vi "LED flashing 1.vi"(0 "Arduino Resource In":T1={"VISA resource"="", "Board Type"=enum."Uno", "Connection Type"=enum."USB / Serial", "Bytes Per Packet (15)"=15}, 11 "Error Out In":errorcluster, 12 "Текущий раствор":i32) -> (1 "1":bool, 2 "2":bool, 3 "3":bool, 4 "Arduino Resource Out":T1={"VISA resource"="", "Board Type"=enum."Uno", "Connection Type"=enum."USB / Serial", "Bytes Per Packet (15)"=15}, 15 "Error Out":errorcluster)   [LabVIEW 2016]
uses:
  <vilib>/LabVIEW Interface for Arduino/Type Defs/Arduino Resource.ctl
  <vilib>/LabVIEW Interface for Arduino/Type Defs/Board Type.ctl
  <vilib>/LabVIEW Interface for Arduino/LabVIEW Interface for Arduino.lvlib
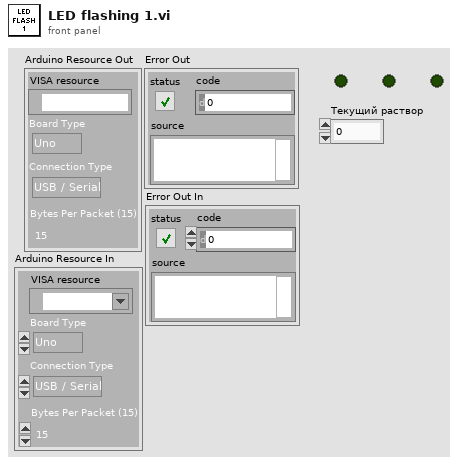
[diagram p1: front panel]
types:
  T1 = typedef "LabVIEW Interface for Arduino.lvlib/Arduino Resource.ctl" = cluster{"VISA resource":refnum<visa-resource-name>, "Board Type":T2, "Connection Type":enum8{"USB / Serial"}, "Bytes Per Packet (15)":u8}
  T2 = typedef "LabVIEW Interface for Arduino.lvlib/Board Type.ctl" = enum16{"Uno", "Dimuelanove w/Atmega 328", "Mega 2560"}
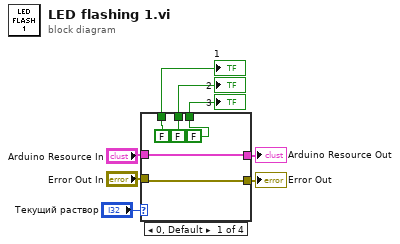
[diagram p0: block diagram]
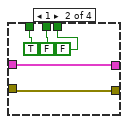
[diagram p2: hidden frame]
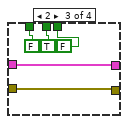
[diagram p3: hidden frame]
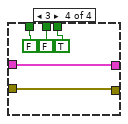
[diagram p4: hidden frame]
diagram:
  n1 = case shown="0, Default" "Текущий раствор" {
    tunnel: "Error Out In" -> [w13 w14 w19 w24]
    tunnel: [w12 w15 w20 w25] -> w2
    tunnel: [w13 w14 w19 w24] -> w1
    tunnel: [FALSE ("3") TRUE ("3") FALSE ("3") FALSE ("3")] -> w8
    tunnel: [FALSE ("3") FALSE ("3") FALSE ("3") TRUE ("3")] -> w7
    tunnel: "Arduino Resource In" -> [w12 w15 w20 w25]
    tunnel: [FALSE ("3") FALSE ("3") TRUE ("3") FALSE ("3")] -> w4
    frame 0, Default {
    }
    frame 1 {
    }
    frame 2 {
    }
    frame 3 {
    }
  }
  "1" <- w8
  "2" <- w4
  "3" <- w7
  "Arduino Resource Out" <- w2
  "Error Out" <- w1
